vi "Is Valid Windows Filename.vi"(8 "error in (no error)":errorcluster, 11 "Filename":string) -> (0 "error out":errorcluster, 1 "empty filename?":bool, 2 "valid windows filename":bool, 3 "appended path":path)   [LabVIEW 2021]
uses:
  <vilib>/Utility/sysdir.llb/System Directory Type.ctl
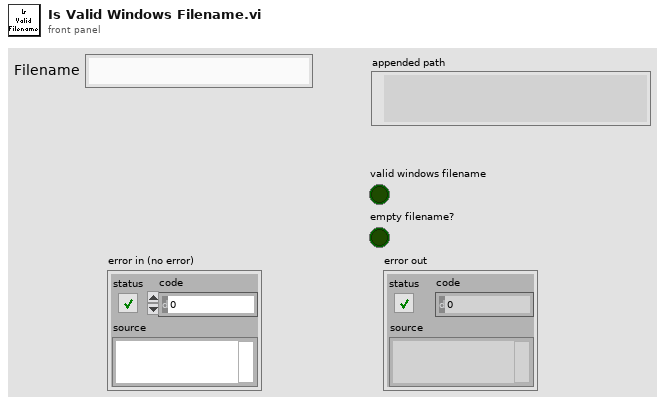
[diagram p1: front panel]
types:
  T1 = enum16{"open", "replace", "create", "open or create", "replace or create", "replace or create with confirmation"}
  T2 = typedef "System Directory Type.ctl" = i32
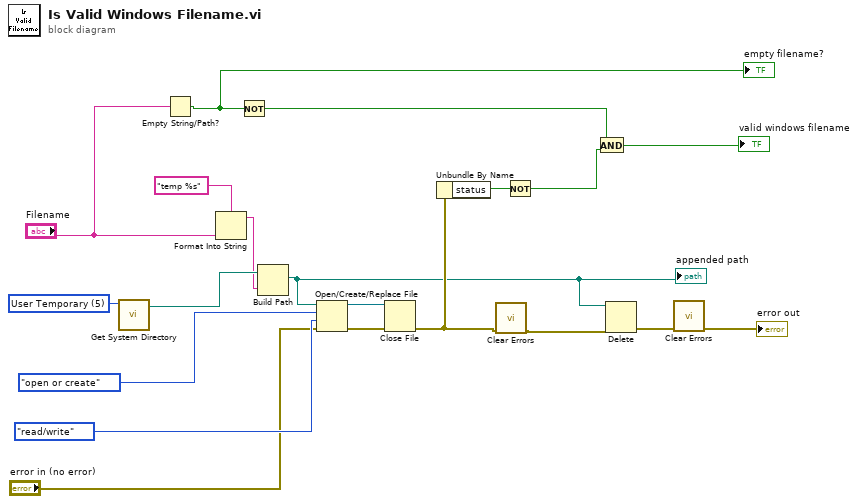
[diagram p0: block diagram]
diagram:
  w20 = T2 5 items=["User Home"=0, "User Desktop"=1, "User Documents"=2, "User Application Data"=3, "User Preferences"=4, "User Temporary"=5, "Public Documents"=6, "Public Application Data"=7, "Public Preferences"=8, "Public Cache"=13, "System Core Libraries"=9, "System Installed Libraries"=10, "Application Files"=11, "Boot Volume Root"=12] ("system directory type")
  n1 = call <vilib>:"Get System Directory.vi"("system directory type"=w20) -> ("system directory"=w18:path)  [unwired: 10 in]
  n2 = Empty String/Path?(string/path="Filename") -> (empty?=w1:bool)
  "empty filename?" <- w1
  n3 = Format Into String(format string="temp %s", "Filename") -> (resulting string=w17:string)  [unwired: 2 in, 1 out]
  n4 = Not(x=w1) -> (.not. x?=w4:bool)
  n5 = Build Path(base path=w18, name or relative path=w17) -> (appended path=w11:path)
  "appended path" <- w11
  n6 = Open/Create/Replace File(file path (use dialog)=w11, error in="error in (no error)", operation (0:open)=T1."open or create", access (0:read/write)=enum16{"read/write", "read-only", "write-only"}."read/write") -> (refnum out=w16:refnum<file>, error out=w15:errorcluster)  [unwired: 2 in, 1 out]
  n7 = Close File(refnum=w16, error in=w15) -> (error out=w13:errorcluster)  [unwired: 1 out]
  n8 = Unbundle By Name(w13) -> ("status"=w14:bool)
  n9 = call <vilib>:"Clear Errors.vi"("error in (no error)"=w13) -> ("error out"=w12:errorcluster)  [unwired: 5 in, 1 out]
  n10 = Not(x=w14) -> (.not. x?=w3:bool)
  n11 = And(x=w4, y=w3) -> (x .and. y?=→"valid windows filename":bool)
  n12 = Delete(path (use dialog)=w11, error in=w12) -> (error out=w10:errorcluster)  [unwired: 3 in, 2 out]
  n13 = call <vilib>:"Clear Errors.vi"("error in (no error)"=w10) -> ("error out"=→"error out":errorcluster)  [unwired: 5 in, 1 out]
